vi "Testx.vi"() -> ()   [LabVIEW 2013]
panel:
  in  "Final Accel Values 3":dbl[][](array[numeric])
  out "Numeric 3":dbl
  out "Numeric 2":dbl
  out "Numeric":dbl
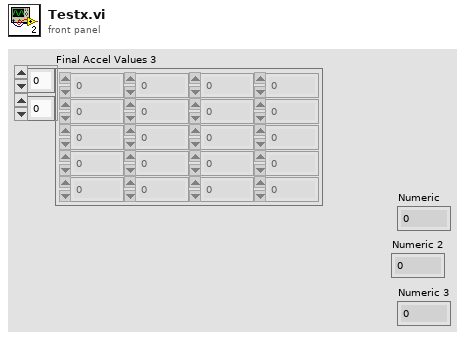
[diagram p1: front panel]
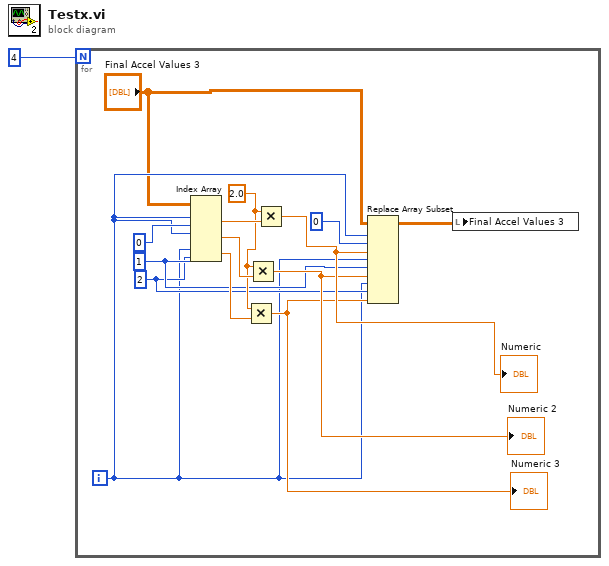
[diagram p0: block diagram]
diagram:
  n1 = for {
    N: 4 -> [_]
    i -> [w4]
    w10 = 2.0
    w5 = 2
    w6 = 1
    n2 = Index Array(array="Final Accel Values 3", index (row) #1=w4, index (col) #1=0, index (row) #2=w4, index (col) #2=w6, index (row) #3=w4, index (col) #3=w5) -> (element #1=w14:dbl, element #2=w12:dbl, element #3=w11:dbl)
    n3 = Multiply(x=w10, y=w11) -> (x*y=w8:dbl)
    "Numeric 3" <- w8
    n4 = Multiply(x=w10, y=w12) -> (x*y=w9:dbl)
    "Numeric 2" <- w9
    n5 = Multiply(x=w10, y=w14) -> (x*y=w13:dbl)
    "Numeric" <- w13
    n6 = Replace Array Subset(array="Final Accel Values 3", new element #1=w13, index (row) #1=w4, index (col) #1=0, new element #2=w9, index (row) #2=w4, index (col) #2=w6, new element #3=w8, index (row) #3=w4, index (col) #3=w5) -> (w2:dbl[][])
    n7 = local write "Final Accel Values 3"(w2) -> ()
  }
